vi "IMAQController.constructor.vi"(0 "name":string, 2 "data in":string, 5 "error in (no error)":errorcluster) -> (14 "i ref out":refnum<vi>, 16 "data out":string, 19 "error out":errorcluster)   [LabVIEW 2014, in "IMAQController.lvlib"]
doc: "This is the constructor of a class.\n\nLicense Agreement for this software:\n\nCopyright (C)\nGesellschaft für Schwerionenforschung, GSI\nPlanckstr. 1\n64291 Darmstadt\nGermany\n\nContact: D.Beck@gsi.de \n\nThis program is free software; you can redistribute it and/or modify it under the terms of the \nGNU General Public License as published by the Free Software Foundation; either version 2 of \nthe license, or (at your option) any later version.\n\nThis program is distributed in the hope that it will be useful, but WITHOUT ANY WARRANTY; \nwithout even the implied warranty of MERCHANTABILITY or FITNESS FOR A PARTICULAR PURPOSE. See the GNU General License for more details (http://www.gnu.org).\n\nGesellschaft für Schwerionenforschung, GSI\nPlanckstr. 1, 64291 Darmstadt, Germany\nFor all questions and ideas contact: M.Richter@gsi.de, H.Brand@gsi.de or D.Beck@gsi.de.\nLast update: 16-JUN-2004"
uses:
  IMAQController.lvlib
  CSCore/CSSystem/CoreLib/CoreLib.string 2 byte array.vi
  CSCore/CSSystem/CoreLib/CoreLib.byte array 2 int.vi
  CSCore/CSSystem/CoreLib/CoreLib.byte array 2 double.vi
  CSCore/CSSystem/CoreLib/CoreLib.byte array 2 string.vi
  CSCore/BaseGUI/BaseGUI.lvlib
  CSCore/CSSystem/CSSystemLib/CSSystemLib.lvlib
  CSCore/BaseProcess/BaseProcess.lvlib
  CSCore/CSObj/CSObj.lvlib
  CSlibraries-extern/DimLVEvent/LVDimInterface/LVDimInterface.lvlib
  CSCore/CSSystem/CoreLib/CoreLib.lvlib
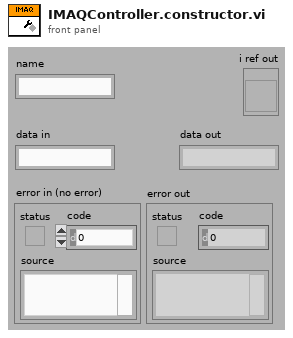
[diagram p1: front panel]
types:
  T1 = enum16{"SetAttribute", "GetAttribute", "CreateAttribute", "DestroyAttribute", "DestroyAllAtributes"}
  T2 = cluster{"Grid":cluster{"1":cluster{i32, i32}, "2":cluster{i32, i32}, "3":cluster{i32, i32}, "4":cluster{i32, i32}}, "GridR":cluster{"1":cluster{dbl, dbl}, "2":cluster{dbl, dbl}, "3":cluster{dbl, dbl}, "4":cluster{dbl, dbl}}}
  T3 = typedef "BaseProcess.lvlib/BaseProcess.i attribute.ctl" = cluster{"EventStatus":string, "EventError":i32, "PresetEvtWatchD":i32, "PresetPdcWatchD":i32, "EventTimeout":i32, "PeriodicInterval":i32, "Interface":string[], "Address":string[], "Special":string[], "PeriodicError":i32, "PeriodicStatus":string, "SuperProc":string, "Descriptors":T4[], "CaseRef":refnum<vi>, "PdcRef":refnum<vi>, "Thread Ref":refnum<vi>, "eventErrorID":i32, "eventStatusID":i32, "periodicErrorID":i32, "periodicStatusID":i32, "pdcCtrID":i32}
  T4 = typedef "BaseProcess.lvlib/BaseProcess.descriptor definition.ctl" = cluster{"selector":string, "descriptor":T5}
  T5 = typedef "BaseProcess.lvlib/BaseProcess.descriptor string definition.ctl" = string
  T6 = typedef "CoreDefs.call_type.ctl" = cluster{"Object":string, "Selector":string, "CallType":enum16{"simple", "synchronous", "asynchronous"}, "Async Object":string, "Async Selector":string, "Data Descriptor":T5, "Data":T7, "Error #":i32, "Expire":u32}
  T7 = typedef "CoreDefs.rawDataType.ctl" = i8[]
  T8 = cluster{"1":cluster{i32, i32}, "2":cluster{i32, i32}, "3":cluster{i32, i32}, "4":cluster{i32, i32}}
  T9 = cluster{"1":cluster{dbl, dbl}, "2":cluster{dbl, dbl}, "3":cluster{dbl, dbl}, "4":cluster{dbl, dbl}}
  T10 = cluster{string, string, u32, bool, dbl, bool, cluster{"i32":i32, "i32":i32}, cluster{"d64":dbl, "d64":dbl}, "d64":dbl, u32, "Grid":cluster{"1":cluster{i32, i32}, "2":cluster{i32, i32}, "3":cluster{i32, i32}, "4":cluster{i32, i32}}, "GridR":cluster{"1":cluster{dbl, dbl}, "2":cluster{dbl, dbl}, "3":cluster{dbl, dbl}, "4":cluster{dbl, dbl}}, dbl, dbl}
  T11 = typedef "IMAQController.lvlib/IMAQController.i attribute.ctl" = cluster{"ImageTakenID":i32, "actSequencer":string, "actScanner":string, "CameraTriggerID":i32, "activatedCameras":cluster{"Name":string, "Camera Type":string, "Acquisition Mode":u32, "JPEG Mode?":bool, "Acquisition Delay":dbl, "Save Images?":bool, "Center Coordinates":T12, "PixelPermm":cluster{"Horizontal":dbl, "Vertical":dbl}, "Rotation":dbl, "Mirror Mode":u32, "PixelCoordinates":cluster{"1":cluster{"Horizontal":i32, "Vertical":i32}, "2":cluster{"Horizontal":i32, "Vertical":i32}, "3":cluster{"Horizontal":i32, "Vertical":i32}, "4":cluster{"Horizontal":i32, "Vertical":i32}}, "RWCoordinates":cluster{"1":cluster{"Horizontal":dbl, "Vertical":dbl}, "2":cluster{"Horizontal":dbl, "Vertical":dbl}, "3":cluster{"Horizontal":dbl, "Vertical":dbl}, "4":cluster{"Horizontal":dbl, "Vertical":dbl}}, "HorizScaling":dbl, "VertScaling":dbl}[], "Ini C-Array":string[], "actCamera":string, "activeCamera":cluster{"Name":string, "Camera Type":string, "Aqcuisation Mode":enum32{"Internal Trigger", "Scan", "free Running", "External Trigger"}, "JPEG Mode?":bool, "Acquisition Delay":dbl, "Save Images?":bool, "Center Coordinates":T12, "PixelPermm":cluster{"Horizontal":dbl, "Vertical":dbl}, "Rotation":dbl, "Mirror Mode":u32, "PixelCoordinates":cluster{"1":cluster{"Horizontal":i32, "Vertical":i32}, "2":cluster{"Horizontal":i32, "Vertical":i32}, "3":cluster{"Horizontal":i32, "Vertical":i32}, "4":cluster{"Horizontal":i32, "Vertical":i32}}, "RWCoordinates":cluster{"1":cluster{"Horizontal":dbl, "Vertical":dbl}, "2":cluster{"Horizontal":dbl, "Vertical":dbl}, "3":cluster{"Horizontal":dbl, "Vertical":dbl}, "4":cluster{"Horizontal":dbl, "Vertical":dbl}}, "HorizScaling":dbl, "VertScaling":dbl}, "BilderMittelungen":u8, "OldPicture":dbl[][]}
  T12 = typedef "LVPoint32TypeDef.ctl" = cluster{"Horizontal":i32, "Vertical":i32}
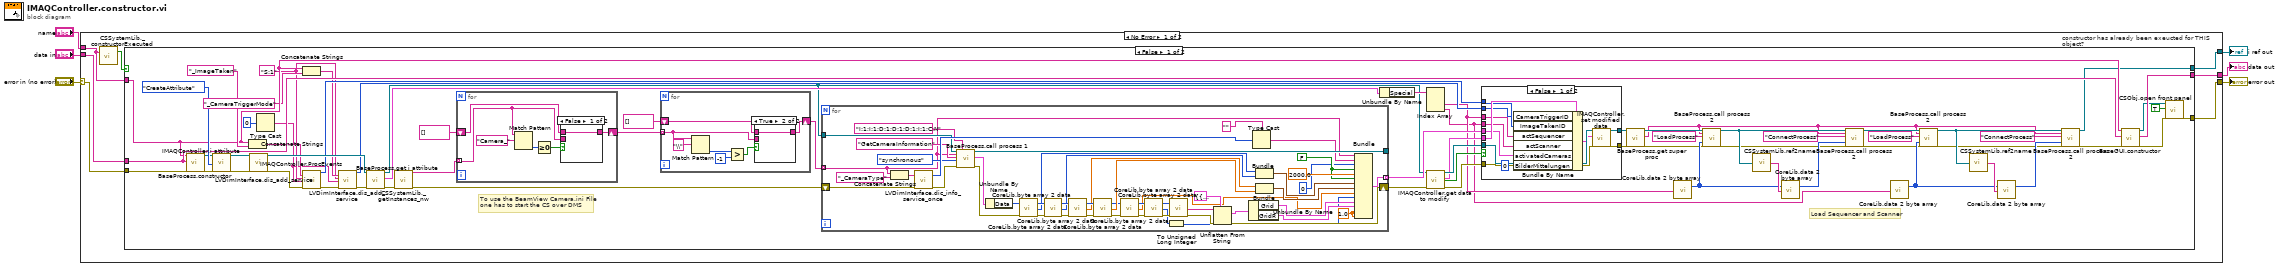
[diagram p0: block diagram]
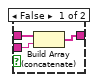
[diagram p2: hidden frame]
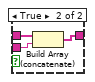
[diagram p3: hidden frame]
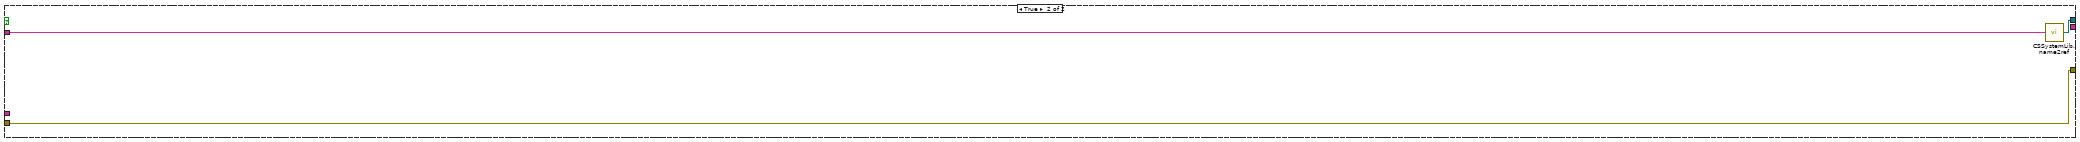
[diagram p5: hidden frame]
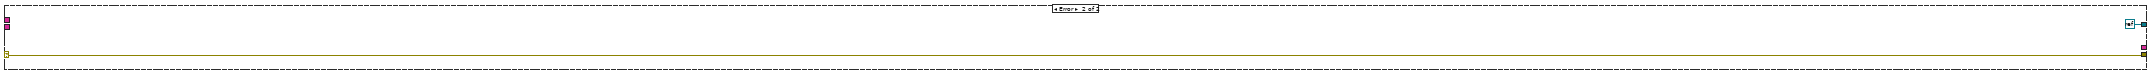
[diagram p6: hidden frame]
diagram:
  n1 = case shown="No Error" "error in (no error)" {
    selector: "error in (no error)" -> [w10 w168]
    tunnel: "data in" -> [w13 _]
    tunnel: "name" -> [w9 _]
    tunnel: [w12 refnum<k0> refnum] -> w4
    tunnel: [w11 w168] -> w3
    tunnel: [w7 _] -> w1
    frame No Error {
      n2 = call "CSSystemLib._constructorExecuted.vi"("name"=w9) -> ("constructor executed?"=w8:bool)  [unwired: 18 in]
      n3 = case "constructor has already been exeucted for THIS object?" shown="False" w8 {
        tunnel: w13 -> [w74 _]
        tunnel: w9 -> [w56 w167]
        tunnel: [w15 w166] -> w12
        tunnel: [w46 w165] -> w11
        tunnel: w10 -> [w77 w165]
        tunnel: [w76 _] -> w7
        frame False {
          w53 = "S:1" ("typeDescriptor")
          # "Load Sequencer and Scanner"
          # "To use the BeamView Camera.ini File\none has to start the CS over DMS"
          n4 = call "BaseProcess.constructor.vi"("name"=w56, "data in"=w74, "error in (no error)"=w77) -> ("i ref out"=w79:refnum<vi>, "error out"=w78:errorcluster)  [unwired: 14 in, 1 out]
          n5 = call "IMAQController.i attribute.vi"("VI Refnum"=w79, "Action"=T1."CreateAttribute", "error in (no error)"=w78) -> ("VI Refnum out"=w72:refnum<vi>, "error out"=w73:errorcluster)  [unwired: 14 in, 1 out]
          n6 = Concatenate Strings(w56, "_ImageTaken" ("string")) -> (w61:string)
          n7 = call "IMAQController.ProcEvents.vi"("i ref in"=w72, "error in (no error)"=w73) -> ("i ref out"=w63:refnum<vi>, "error out"=w64:errorcluster)  [unwired: 16 in]
          n8 = Type Cast(x=i16 0) -> (*(type *) &x=w52:string)  [unwired: 1 in]
          n9 = Concatenate Strings(w56, "_CameraTriggerMode" ("string")) -> (w54:string)
          n10 = call "LVDimInterface.dis_add_service.vi"("serviceName"=w61, "typeDescriptor"=w53, "data"=w52, "error in (no error)"=w64) -> ("my_serviceID"=w60:i32, "error out"=w59:errorcluster)  [unwired: 14 in]
          n11 = call "LVDimInterface.dis_add_service.vi"("serviceName"=w54, "typeDescriptor"=w53, "data"=w52, "error in (no error)"=w59) -> ("my_serviceID"=w57:i32, "error out"=w58:errorcluster)  [unwired: 14 in]
          n12 = call "BaseProcess.get i attribute.vi"("i ref in"=w63, "error in (no error)"=w58) -> ("i ref out"=w39:refnum<vi>, "i attribute"=w67:T3, "error out"=w47:errorcluster)  [unwired: 15 in]
          n13 = call "CSSystemLib._getInstances_nw.vi"("error in (no error)"=w47) -> ("i list"=w48:string[], "error out"=w42:errorcluster)  [unwired: 17 in]
          n14 = for {
            tunnel: w48 -> [w141] mode=indexing
            shift-right: [w143] -> w45
            shift-left: string[] [] -> [w142]
            n15 = Match Pattern(string=w141, regular expression="Camera_") -> (offset past match=w145:i32)  [unwired: 1 in, 3 out]
            n16 = Greater Or Equal To 0?(x=w145) -> (x >= 0?=w144:bool)
            n17 = case shown="False" w144 {
              tunnel: [w147 w150] -> w143
              tunnel: w142 -> [w147 w149]
              tunnel: w141 -> [_ w148]
              frame False {
              }
              frame True {
                n18 = Build Array (concatenate)(w149, w148) -> (w150:string[])
              }
            }
          }
          n19 = for {
            tunnel: w45 -> [w82] mode=indexing
            shift-right: [w81] -> w43
            shift-left: string[] [] -> [w83]
            n20 = Match Pattern(string=w82, regular expression="\\") -> (offset past match=w86:i32)  [unwired: 1 in, 3 out]
            n21 = Greater?(x=w86, y=-1) -> (0:w84:bool)
            n22 = case shown="True" w84 {
              tunnel: w83 -> [w89 w91]
              tunnel: [w90 w91] -> w81
              tunnel: w82 -> [w88 _]
              frame False {
                n23 = Build Array (concatenate)(w89, w88) -> (w90:string[])
              }
              frame True {
              }
            }
          }
          n24 = for {
            tunnel: w43 -> [w116] mode=indexing
            shift-right: [w117] -> w50
            shift-left: w42 -> [w137]
            tunnel: w39 -> [w135]
            tunnel: [w134] -> _
            tunnel: [w105] -> w49 mode=indexing
            w104 = 1.0
            w113 = FALSE
            n25 = Concatenate Strings(w116, "_CameraType" ("string")) -> (w140:string)
            n26 = call "LVDimInterface.dic_info_service_once.vi"("serviceName"=w140, "error in (no error)"=w137) -> ("data"=w139:i8[], "error out"=w133:errorcluster)  [unwired: 14 in, 2 out]
            n27 = call "BaseProcess.call process 1.vi"("i ref in"=w135, "Object"=w116, "Selector"="GetCameraInformation", "CallType"=enum16{"simple", "synchronous", "asynchronous"}."synchronous", "error in (no error)"=w133, "Data Descriptor"="I:1;I:1;D:1;D:1;D:1;I:1;C:N") -> ("i ref out"=w134:refnum<vi>, "call cluster out"=w124:T6, "error out"=w122:errorcluster)  [unwired: 11 in]
            n28 = Unbundle By Name(w124) -> ("Data"=w123:T7)
            n29 = call-poly "CoreLib.byte array 2 data.vi"("byteArray"=w123, "error in (no error)"=w122) -> ("byteArray out"=w125:T7, "i32"=w112:i32, "error out"=w121:errorcluster)  [unwired: 15 in]
            n30 = call-poly "CoreLib.byte array 2 data.vi"("byteArray"=w125, "error in (no error)"=w121) -> ("byteArray out"=w126:T7, "i32"=w111:i32, "error out"=w120:errorcluster)  [unwired: 15 in]
            n31 = call-poly "CoreLib.byte array 2 data.vi"("byteArray"=w126, "error in (no error)"=w120) -> ("byteArray out"=w127:T7, "d64"=w103:dbl, "error out"=w119:errorcluster)  [unwired: 15 in]
            n32 = call-poly "CoreLib.byte array 2 data.vi"("byteArray"=w127, "error in (no error)"=w119) -> ("byteArray out"=w93:T7, "d64"=w102:dbl, "error out"=w94:errorcluster)  [unwired: 15 in]
            n33 = call-poly "CoreLib.byte array 2 data.vi"("byteArray"=w93, "error in (no error)"=w94) -> ("byteArray out"=w96:T7, "d64"=w92:dbl, "error out"=w95:errorcluster)  [unwired: 15 in]
            n34 = call-poly "CoreLib.byte array 2 data.vi"("byteArray"=w96, "error in (no error)"=w95) -> ("byteArray out"=w99:T7, "i32"=w98:i32, "error out"=w100:errorcluster)  [unwired: 15 in]
            n35 = To Unsigned Long Integer(number=w98) -> (unsigned 32bit integer=w97:u32)
            n36 = call-poly "CoreLib.byte array 2 data.vi"("byteArray"=w99, "error in (no error)"=w100) -> ("string"=w128:string, "error out"=w118:errorcluster)  [unwired: 15 in, 1 out]
            n37 = Unflatten From String(type=T2 {"Grid"={"1"={0, 0}, "2"={0, 0}, "3"={0, 0}, "4"={0, 0}}, "GridR"={"1"={0.0, 0.0}, "2"={0.0, 0.0}, "3"={0.0, 0.0}, "4"={0.0, 0.0}}} ("output cluster"), binary string=w128, error in (no error)=w118) -> (value=w108:T2, error out=w117:errorcluster)  [unwired: 2 in, 1 out]
            n38 = Unbundle By Name(w108) -> ("Grid"=w107:T8, "GridR"=w106:T9)
            n39 = Type Cast(type="", x=w139) -> (*(type *) &x=w115:string)
            n40 = Bundle("i32"=w112, "i32"=w111) -> (w110:cluster{"i32":i32, "i32":i32})  [unwired: 1 in]
            n41 = Bundle("d64"=w103, "d64"=w102) -> (w101:cluster{"d64":dbl, "d64":dbl})  [unwired: 1 in]
            n42 = Bundle(w116, w115, u32 0, w113, 2000.0, w113, w110, w101, "d64"=w92, w97, "Grid"=w107, "GridR"=w106, w104, w104) -> (w105:T10)  [unwired: 1 in]
          }
          n43 = Unbundle By Name(w67) -> ("Special"=w66:string[])
          n44 = Index Array(array=w66) -> (element #2=w27:string, element #3=w16:string)  [unwired: 3 in, 1 out]
          n45 = call "IMAQController.get data to modify.vi"("i ref in"=w39, "error in (no error)"=w50) -> ("i ref out"=w69:refnum<vi>, "i attribute"=w68:T11, "timed out"=w71:bool, "error out"=w70:errorcluster)  [unwired: 14 in]
          n46 = case shown="False" w71 {
            tunnel: w70 -> [w162 w164]
            tunnel: [w161 w164] -> w30
            tunnel: w69 -> [w160 w163]
            tunnel: [w159 w163] -> w31
            tunnel: w68 -> [w158 _]
            tunnel: w27 -> [w156 _]
            tunnel: w16 -> [w155 _]
            tunnel: w60 -> [w154 _]
            tunnel: w57 -> [w153 _]
            tunnel: w49 -> [w152 _]
            frame False {
              n47 = Bundle By Name(cluster=w158, "CameraTriggerID"=w153, "ImageTakenID"=w154, "actSequencer"=w156, "actScanner"=w155, "activatedCameras"=w152, "BilderMittelungen"=u8 0) -> (w157:T11)
              n48 = call "IMAQController.set modified data.vi"("i ref in"=w160, "i attribute"=w157, "error in (no error)"=w162) -> ("i ref out"=w159:refnum<vi>, "error out"=w161:errorcluster)  [unwired: 15 in]
            }
            frame True {
            }
          }
          n49 = call "BaseProcess.get super proc.vi"("i ref in"=w31, "error in (no error)"=w30) -> ("i ref out"=w29:refnum<vi>, "SuperProc"=w17:string, "error out"=w28:errorcluster)  [unwired: 15 in]
          n50 = call-poly "CoreLib.data 2 byte array.vi"("string"=w27) -> ("byteArray out"=w33:T7)  [unwired: 18 in]
          n51 = call "BaseProcess.call process 2.vi"("i ref in"=w29, "Object"=w17, "Selector"="LoadProcess", "Data"=w33, "error in (no error)"=w28) -> ("i ref out"=w35:refnum<vi>, "error out"=w32:errorcluster)  [unwired: 13 in]
          n52 = call "CSSystemLib.ref2name.vi"("obj refnum"=w35) -> ("name"=w37:string)
          n53 = call-poly "CoreLib.data 2 byte array.vi"("byteArray"=w33, "string"=w37) -> ("byteArray out"=w36:T7)  [unwired: 17 in]
          n54 = call "BaseProcess.call process 2.vi"("i ref in"=w35, "Object"=w17, "Selector"="ConnectProcess", "Data"=w36, "error in (no error)"=w32) -> ("i ref out"=w19:refnum<vi>, "error out"=w18:errorcluster)  [unwired: 13 in]
          n55 = call-poly "CoreLib.data 2 byte array.vi"("string"=w16) -> ("byteArray out"=w21:T7)  [unwired: 18 in]
          n56 = call "BaseProcess.call process 2.vi"("i ref in"=w19, "Object"=w17, "Selector"="LoadProcess", "Data"=w21, "error in (no error)"=w18) -> ("i ref out"=w23:refnum<vi>, "error out"=w20:errorcluster)  [unwired: 13 in]
          n57 = call "CSSystemLib.ref2name.vi"("obj refnum"=w23) -> ("name"=w25:string)
          n58 = call-poly "CoreLib.data 2 byte array.vi"("byteArray"=w21, "string"=w25) -> ("byteArray out"=w24:T7)  [unwired: 17 in]
          n59 = call "BaseProcess.call process 2.vi"("i ref in"=w23, "Object"=w17, "Selector"="ConnectProcess", "Data"=w24, "error in (no error)"=w20) -> ("i ref out"=w15:refnum<vi>, "error out"=w14:errorcluster)  [unwired: 13 in]
          n60 = call "BaseGUI.constructor.vi"("name"=w56, "data in"=w74, "error in (no error)"=w14) -> ("i ref out"=w41:refnum<vi>, "data out"=w76:string, "error out"=w40:errorcluster)  [unwired: 14 in]
          n61 = call "CSObj.open front panel.vi"("i ref in"=w41, "frontPanelOpen"=TRUE ("front panel open"), "error in (no error)"=w40) -> ("error out"=w46:errorcluster)  [unwired: 15 in, 1 out]
        }
        frame True {
          n62 = call "CSSystemLib.name2ref.vi"("name"=w167) -> ("obj refnum"=w166:refnum<vi>)
        }
      }
    }
    frame Error {
    }
  }
  "i ref out" <- w4
  "error out" <- w3
  "data out" <- w1
